vi "Assoc.vi"() -> ()   [LabVIEW 2021]
uses:
  Expression.ctl
  ExpressionType.ctl
  Environment.ctl
panel:
  in  "Environment":T1
  out "Expression out":T2
  in  "Expression in":T2
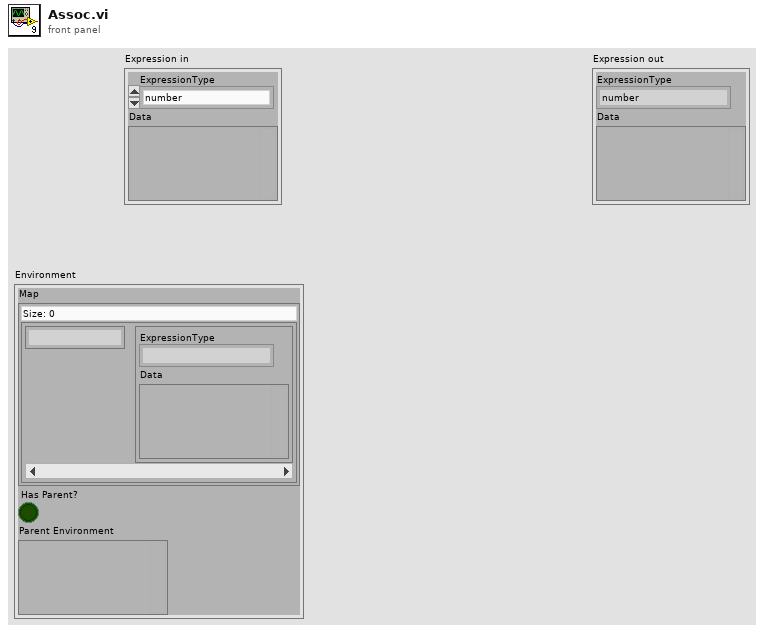
[diagram p1: front panel]
types:
  T1 = typedef "Environment.ctl" = cluster{"Map":map{string, T2}, "Has Parent?":bool, "Parent Environment":variant}
  T2 = typedef "Expression.ctl" = cluster{"ExpressionType":T3, "Data":variant}
  T3 = typedef "ExpressionType.ctl" = enum16{"number", "string", "symbol", "primitive", "list", "closure", "nil", "error"}
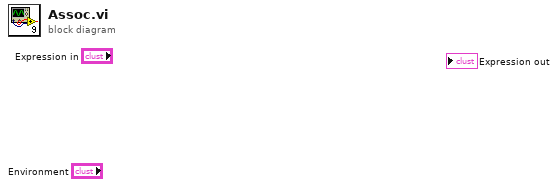
[diagram p0: block diagram]
diagram:
